vi "XML Parse Boolean.vi"(3 "Attribut Name":string, 7 "XML Response":string) -> (0 "Wert (boolean)":bool, 2 "XML Response gekürzt":string)   [LabVIEW 2020, in "FT-IR.lvlib" / "TOOLweb Interface.lvlib" / "TOOLweb Interface Hilfs-VIs.lvlib"]
doc: "Sucht in dem XML-Poll-Response-String \"XML-Response\" den Eintrag mit dem Elementnamen \"Attribut Name\" und liefert dessen Wert in \"Wert (boolean)\". \n\nDer Eintrag wird dann entfernt, damit eine weiteres Parser-VI am Ausgang \"XML Response gekürzt\" nicht wieder den ganzen String durchsuchen muss."
uses:
  TOOLweb Interface Hilfs-VIs.lvlib
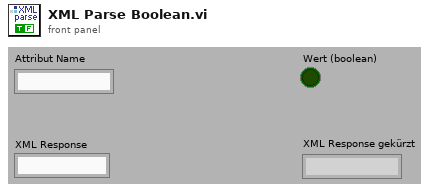
[diagram p1: front panel]
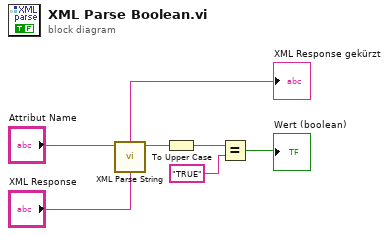
[diagram p0: block diagram]
diagram:
  n1 = call "XML Parse String.vi"("Attribut Name"="Attribut Name", "XML Response"="XML Response") -> ("Wert-String"=w4:string, "XML Response gekürzt"=→"XML Response gekürzt":string)  [unwired: 6 out]
  n2 = To Upper Case(1:w4) -> (0:w3:string)
  n3 = Equal?(x=w3, y="TRUE") -> (x = y?=→"Wert (boolean)":bool)
